vi "AO Continuous Smart Write.vi"(4 "Wait Until Done?":bool, 6 "Stop?":bool, 7 "Data To Write":dbl[][](array[numeric]), 8 "error in (no error)":errorcluster, 9 "Timeout":i32=-1 min=-1, 10 "Sample Rate":dbl=1000.0 min=1000.0 max=30000.0, 11 "Channel Names":tag[](array[tag])) -> (0 "error out":errorcluster)   [LabVIEW 2021, in "AO Continuous.lvlib"]
uses:
  <vilib>/myRIO/Instrument Drivers/Onboard IO/AO Continuous/AO Continuous.lvlib
  <vilib>/userdefined/High Color/nirio_resource_hc.ctl
  <vilib>/myRIO/Common/Instrument Driver Framework/Utilities/typedefs/Hardware Version Enum.ctl
  <vilib>/myRIO/Instrument Drivers/Onboard IO/AO Continuous/typedefs/AO Continuous Reference.ctl
  <vilib>/myRIO/Common/Instrument Driver Framework/Utilities/typedefs/myRIO Generic Hardware Reference.ctl
  <vilib>/myRIO/Common/Instrument Driver Framework/Utilities/typedefs/myRIO v1.0 Reference.ctl
  <vilib>/myRIO/Common/Instrument Driver Framework/Utilities/typedefs/Generic FPGA Reference.ctl
  <vilib>/myRIO/Common/Instrument Driver Framework/ELVIS III v1.0/AO Continuous/typedefs/AO Continuous Channels List.ctl
  <vilib>/myRIO/Common/Instrument Driver Framework/ELVIS III v1.0/AO Continuous/typedefs/ELVIS III v1.0 AO Continuous Channels Enum.ctl
  <vilib>/myRIO/Common/Instrument Driver Framework/ELVIS III v1.0/AO Continuous/typedefs/AO Continuous Channel Info.ctl
  <vilib>/myRIO/Common/Instrument Driver Framework/ELVIS III v1.0/AO Continuous/vis/ELVIS III v1.1 Open AO (Continuous).vi
  <vilib>/myRIO/Common/Instrument Driver Framework/Utilities/vis/Validate Channels.vi
  <vilib>/myRIO/Common/Instrument Driver Framework/ELVIS III v1.0/AO Continuous/vis/ELVIS III v1.0 Reserve AO Continuous.vi
  <vilib>/myRIO/Common/Instrument Driver Framework/ELVIS III v1.0/AO Continuous/vis/ELVIS III v1.0 Build MUX Configuration AO Continuous.vi
  <vilib>/Utility/error.llb/Error Cluster From Error Code.vi
  <vilib>/Utility/VariantDataType/GetNumericInfo.vi
  <vilib>/myRIO/Common/Instrument Driver Framework/ELVIS III v1.0/ELVIS III v1.1 Open.vi
  <vilib>/myRIO/Common/Instrument Driver Framework/ELVIS III v1.0/Resource Manager/vis/ELVIS III v1.0 Reserve Channel List.vi
  <vilib>/myRIO/Common/Instrument Driver Framework/ELVIS III v1.0/Resource Manager/vis/ELVIS III v1.0 Configure DMAs.vi
  <vilib>/myRIO/Common/Instrument Driver Framework/myRIO v1.0/myRIO v1.0 Close.vi
  <vilib>/myRIO/Common/Instrument Driver Framework/ELVIS III v1.0/AO Continuous/vis/ELVIS III v1.1 Stop AO Continuous.vi
  <vilib>/myRIO/Instrument Drivers/Onboard IO/AO Continuous/vis/myRIO AO Continuous Open.xnode
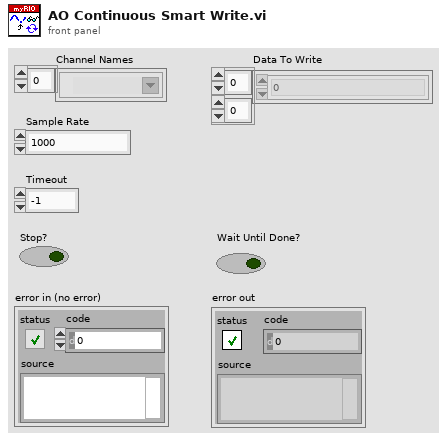
[diagram p1: front panel]
types:
  T1 = typedef "nirio_resource_hc.ctl" = tag
  T2 = typedef "Hardware Version Enum.ctl" = enum16{"Unknown", "myRIO-1900", "myRIO-1950", "roboRIO", "NI ELVIS RIO CM", "ELVIS III"}
  T3 = typedef "AO Continuous.lvlib/AO Continuous Reference.ctl" = cluster{"myRIO Reference":T4, "AO (Continuous) Channels List":T7, "Channel Info":T9}
  T4 = typedef "myRIO Generic Hardware Reference.ctl" = cluster{"myRIO Model":T2, "myRIO Hardware Reference":T5}
  T5 = typedef "myRIO v1.0 Reference.ctl" = cluster{"Generic FPGA Reference":T6, "Allow multiple opens":bool}
  T6 = typedef "Generic FPGA Reference.ctl" = refnum<k20>
  T7 = typedef "AO Continuous Channels List.ctl" = T8[]
  T8 = typedef "ELVIS III v1.0 AO Continuous Channels Enum.ctl" = enum16{"Not Connected", "A/AO0 (Continuous)", "A/AO1 (Continuous)", "B/AO0 (Continuous)", "B/AO1 (Continuous)"}
  T9 = typedef "AO Continuous Channel Info.ctl" = cluster{"Channel Bitmask":u8[], "Channel Index":i32[], "Channel Number":u8}
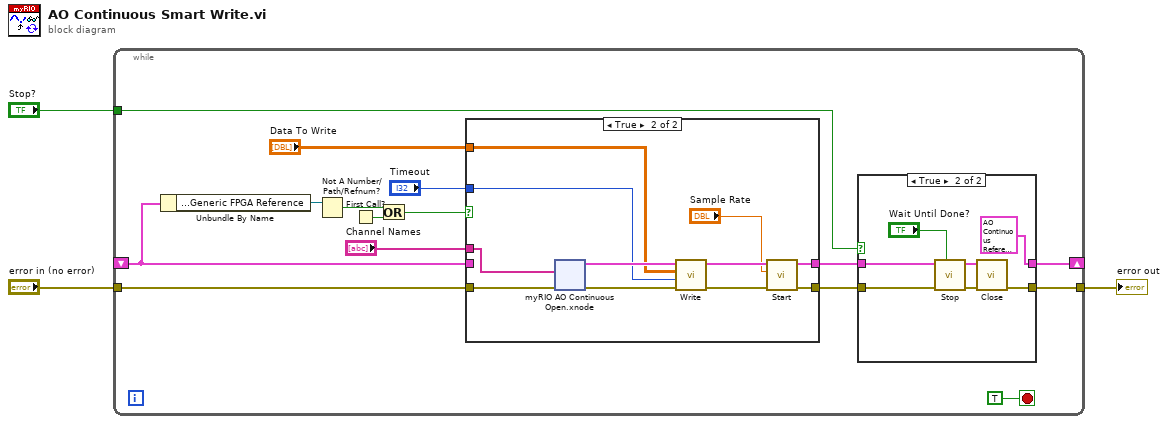
[diagram p0: block diagram]
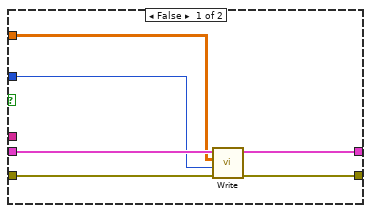
[diagram p2: hidden frame]
diagram:
  n1 = while {
    tunnel: [w17] -> w3
    tunnel: "error in (no error)" -> [w16]
    shift-right: [w14] -> _
    shift-left: _ -> [w13]
    tunnel: "Stop?" -> [w8]
    stop <- TRUE stop-if-true
    n2 = Unbundle By Name(w13) -> ("myRIO Reference.myRIO Hardware Reference.Generic FPGA Reference"=w10:T6)
    n3 = Not A Number/Path/Refnum?(number/path/refnum=w10) -> (NaN/Path/Refnum?=w9:bool)
    n4 = First Call?() -> (First Call?: T/F=w12:bool)
    n5 = Or(x=w9, y=w12) -> (x .or. y?=w11:bool)
    n6 = case shown="True" w11 {
      tunnel: "Channel Names" -> [_ w35]
      tunnel: [w21 w29] -> w5
      tunnel: [w22 w28] -> w6
      tunnel: w16 -> [w24 w27]
      tunnel: w13 -> [w23 _]
      tunnel: "Data To Write" -> [w20 w26]
      tunnel: "Timeout" -> [w19 w25]
      frame False {
        n7 = call <vilib>:"Write.vi"("error in (no error)"=w24, "Timeout"=w19, "Data To Write"=w20, "AO (Continuous) Ref In"=w23) -> ("error out"=w21:errorcluster, "AO (Continuous) Ref Out"=w22:T3)  [unwired: 6 in]
      }
      frame True {
        n8 = xnode "myRIO AO Continuous Open.xnode"("error in (no error)"=w27, "Channel Names"=w35) -> ("error out"=w33:errorcluster, "AO (Continuous) Ref Out"=w34:T3)
        n9 = call <vilib>:"Write.vi"("error in (no error)"=w33, "Timeout"=w25, "Data To Write"=w26, "AO (Continuous) Ref In"=w34) -> ("error out"=w32:errorcluster, "AO (Continuous) Ref Out"=w31:T3)  [unwired: 6 in]
        n10 = call <vilib>:"Start.vi"("error in (no error)"=w32, "Sample Rate"="Sample Rate", "AO (Continuous) Ref In"=w31) -> ("error out"=w29:errorcluster, "AO (Continuous) Ref Out"=w28:T3)  [unwired: 7 in]
      }
    }
    n11 = case shown="True" w8 {
      tunnel: w5 -> [w53 w61]
      tunnel: w6 -> [w54 w60]
      tunnel: [w53 w56] -> w17
      tunnel: [w54 T3 {"myRIO Reference"={"myRIO Model"=enum."Unknown", "myRIO Hardware Reference"={"Generic FPGA Reference"=refnum, "Allow multiple opens"=FALSE}}, "AO (Continuous) Channels List"=[], "Channel Info"={"Channel Bitmask"=[], "Channel Index"=[], "Channel Number"=0}} ("AO (Continuous) Ref Out")] -> w14
      frame False {
      }
      frame True {
        n12 = call <vilib>:"Stop.vi"("Wait Until Done?"="Wait Until Done?", "error in (no error)"=w61, "AO (Continuous) Ref In"=w60) -> ("error out"=w59:errorcluster, "AO (Continuous) Ref Out"=w58:T3)  [unwired: 7 in]
        n13 = call <vilib>:"Close.vi"("error in (no error)"=w59, "AO (Continuous) Ref In"=w58) -> ("error out"=w56:errorcluster)  [unwired: 9 in]
      }
    }
  }
  "error out" <- w3
